vi "_unittest Add Test Case.vi"(8 "error in (no error)":errorcluster, 11 "Test Case":string) -> (0 "error out":errorcluster)   [LabVIEW 2019, in "labview_json_tests.lvlib"]
uses:
  labview_json_tests.lvlib
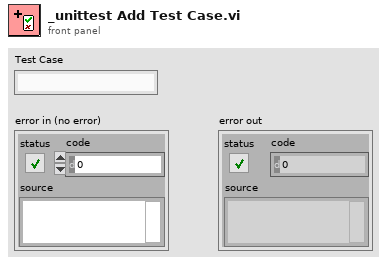
[diagram p1: front panel]
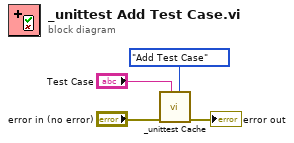
[diagram p0: block diagram]
diagram:
  n1 = call "_unittest Cache.vi"("Action"=enum8{"Report", "Add Test Case", "Add Test"}."Add Test Case", "Message"="Test Case", "error in (no error)"="error in (no error)") -> ("error out"=→"error out":errorcluster)  [unwired: 7 in, 1 out]
